vi "test fp.vi"() -> ()   [LabVIEW 2020]
panel:
  in  "exit":bool
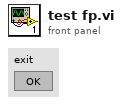
[diagram p1: front panel]
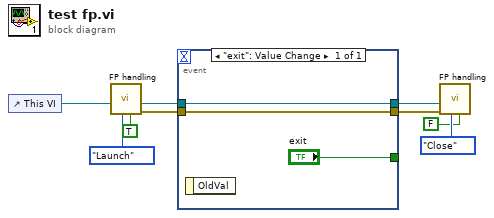
[diagram p0: block diagram]
diagram:
  n1 = control-ref of="This VI"() -> (w8:refnum<vi>)
  n2 = call "FP handling.vi"("initial"=TRUE, "State"=enum16{"Launch", "Close"}."Launch", "VI in"=w8) -> ("error out"=w9:errorcluster, "VI out"=w7:refnum<vi>)  [unwired: 7 in]
  n3 = event shown="[0] \"exit\": Value Change" {
    selector: _ -> [_]
    dyn-events: _ -> [_]
    timeout: _ -> [_]
    tunnel: ["exit"] -> _
    tunnel: w9 -> [w11]
    tunnel: [w11] -> w5
    tunnel: [w10] -> w6
    tunnel: w7 -> [w10]
    event "exit": Value Change {
      n4 = event-data() -> ()  [unwired: 1 in, 1 out]
    }
  }
  n5 = call "FP handling.vi"("initial"=FALSE, "State"=enum16{"Launch", "Close"}."Close", "error in (no error)"=w5, "VI in"=w6) -> ()  [unwired: 6 in, 2 out]
